vi "fgv_txtfile.vi"(7 "cmd":enum16{"write", "create"}(ring), 8 "err in":errorcluster) -> (0 "error out":errorcluster caption="err out")   [LabVIEW 2016]
uses:
  <vilib>/Utility/file.llb/Write To Spreadsheet File (string).vi
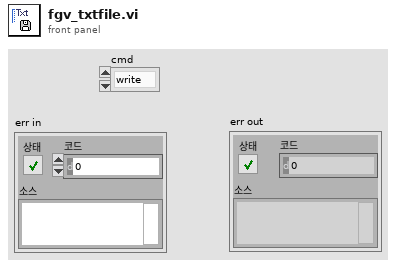
[diagram p1: front panel]
types:
  T1 = enum16{"open", "replace", "create", "open or create", "replace or create", "replace or create with confirmation"}
  T2 = typedef "Total data.ctl" = cluster{"Raw Data":T3, "Resister result data":T4, "Result Table update":cluster{"Num":u32[], "Resister 1~5":u8[][], "Resister 6~10":u8[][], "Resister 11~15":u8[][]}, "Strain Data":cluster{"Strain 1":dbl, "Strain 2":dbl, "Strain 3":dbl, "Strain 4":dbl}, "Acc Result":cluster{"Acc Peak":dbl, "Acc time":dbl, "Acc area":dbl}, "STATUS":cluster{"status":string, "all_fail":bool, "emg":bool, "cycle":u16, "file name":string}, "Speed":dbl, "Acc peak time":dbl, "Max Strain":dbl, "Resistor at peak":cluster{"[0]":dbl, "[1]":dbl, "[2]":dbl, "[3]":dbl, "[4]":dbl, "[5]":dbl, "[6]":dbl, "[7]":dbl, "[8]":dbl, "[9]":dbl, "[10]":dbl, "[11]":dbl, "[12]":dbl, "[13]":dbl, "[14]":dbl}, "Acc peak index":u32, "time":string, "Cycle finish":bool, "Resistor at ini":cluster{"[0]":dbl, "[1]":dbl, "[2]":dbl, "[3]":dbl, "[4]":dbl, "[5]":dbl, "[6]":dbl, "[7]":dbl, "[8]":dbl, "[9]":dbl, "[10]":dbl, "[11]":dbl, "[12]":dbl, "[13]":dbl, "[14]":dbl}}
  T3 = typedef "raw Q data.ctl" = cluster{"Res_data":waveform(dbl)[], "Acc_data":waveform(dbl), "Strain_data":waveform(dbl)[]}
  T4 = typedef "raw data type.ctl" = cluster{"Resistor values":cluster{"[0]":dbl, "[1]":dbl, "[2]":dbl, "[3]":dbl, "[4]":dbl, "[5]":dbl, "[6]":dbl, "[7]":dbl, "[8]":dbl, "[9]":dbl, "[10]":dbl, "[11]":dbl, "[12]":dbl, "[13]":dbl, "[14]":dbl}, "Resistor tables":u8[], "Pass Fails":bool[]}
  T5 = cluster{"Strain 1":dbl, "Strain 2":dbl, "Strain 3":dbl, "Strain 4":dbl}
  T6 = cluster{"[0]":dbl, "[1]":dbl, "[2]":dbl, "[3]":dbl, "[4]":dbl, "[5]":dbl, "[6]":dbl, "[7]":dbl, "[8]":dbl, "[9]":dbl, "[10]":dbl, "[11]":dbl, "[12]":dbl, "[13]":dbl, "[14]":dbl}
  T7 = cluster{"Test Information":cluster{"date":string, "custom":string, "oper":string, "package":string, "pkg side":string, "solder":string, "brd side":string, "paste":string, "reflow":string}, "Sensor Set":cluster{"Accelerometer":cluster{"Sensitivity(mV/g)":dbl}, "Strain Guage":cluster{"Ch.":dbl[], "Gage factor":dbl[], "Resistance":dbl[], "Poisson ratio":dbl[]}}, "Resistor Set":cluster{"Criterion Level":dbl, "Res. Set":cluster{"Res. Ch":dbl, "Res. Active":bool, "Res Initial":dbl}[]}, "Test Stop Condition":cluster{"Test cycle":u16, "Fail number in a cycle":u16, "Fail factor":cluster{"Duration":u16, "Fail No.":u16}}, "Acceleration Condition ":cluster{"Shock duration pecent [%]":u16, "Filter cutoff freq":u32}, "Save":cluster{"Save Path":path, "File Name":string}}
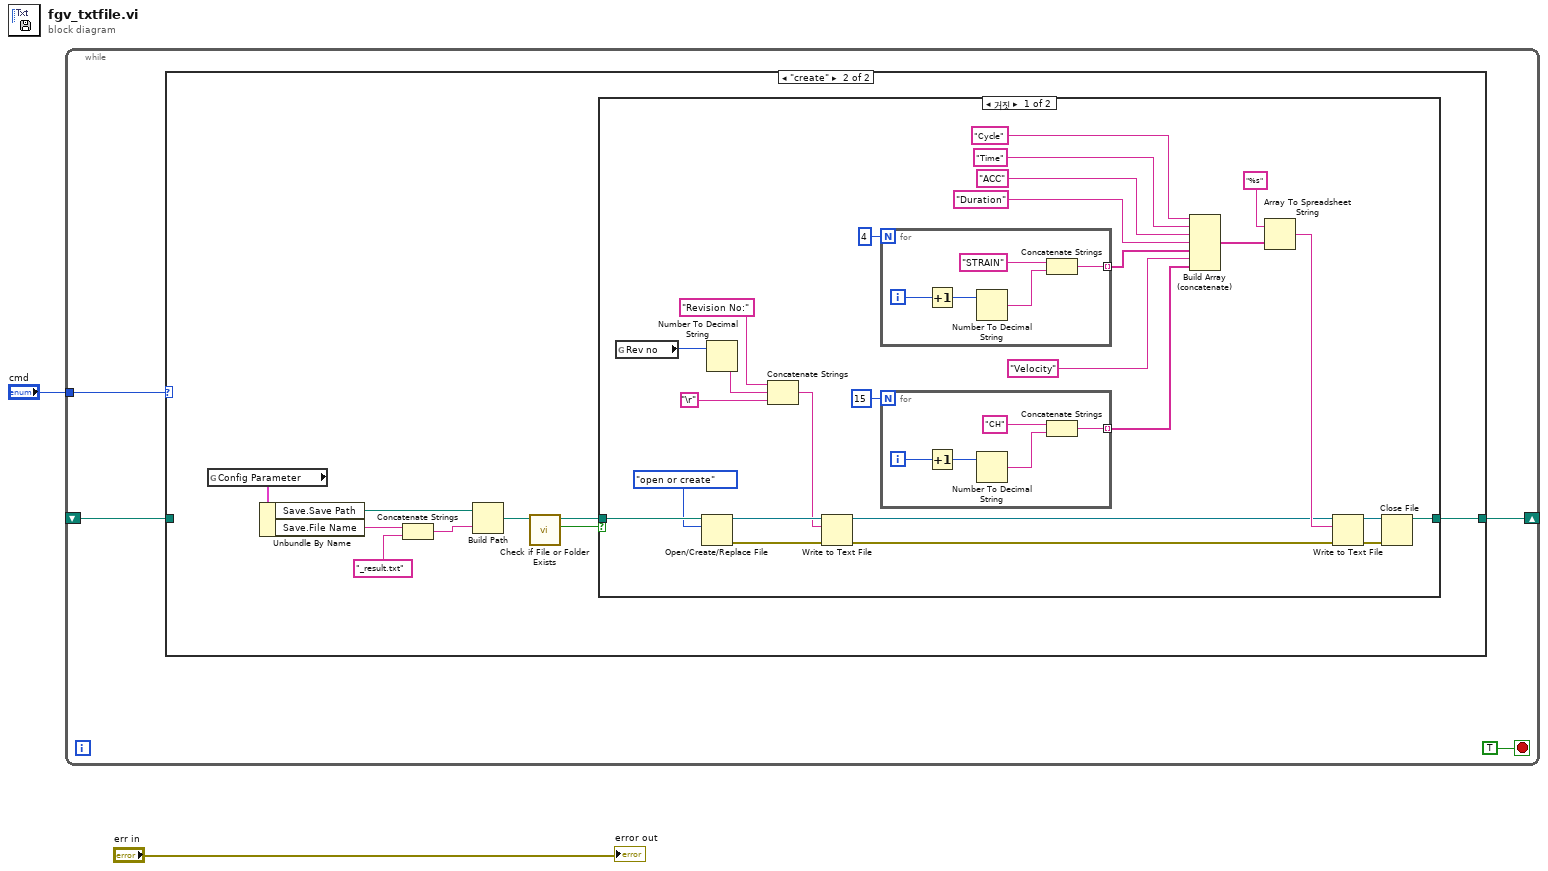
[diagram p0: block diagram]
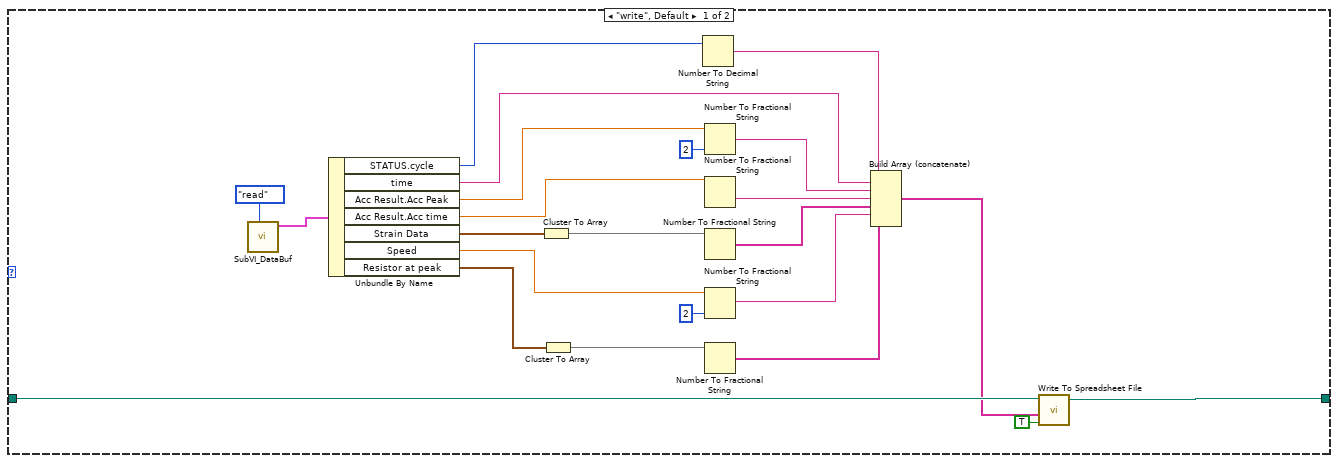
[diagram p2: hidden frame]
diagram:
  n1 = while {
    tunnel: "cmd" -> [w5]
    shift-right: [w4] -> _
    shift-left: _ -> [w3]
    stop <- TRUE stop-if-true
    n2 = case shown="\"create\"" w5 {
      tunnel: [w28 w30] -> w4
      tunnel: w3 -> [w25 _]
      frame "write", Default {
        n3 = call "SubVI_DataBuf.vi"("cmd"=enum16{"ini", "write", "read"}."read") -> ("Total data 2"=w27:T2)  [unwired: 9 in, 1 out]
        n4 = Unbundle By Name(w27) -> ("STATUS.cycle"=w24:u16, "time"=w7:string, "Acc Result.Acc Peak"=w23:dbl, "Acc Result.Acc time"=w9:dbl, "Strain Data"=w21:T5, "Speed"=w11:dbl, "Resistor at peak"=w13:T6)
        n5 = Cluster To Array(cluster=w21) -> (array=w20:dbl[])
        n6 = Cluster To Array(cluster=w13) -> (array=w19:dbl[])
        n7 = Number To Decimal String(number=w24) -> (decimal integer string=w18:string)  [unwired: 1 in]
        n8 = Number To Fractional String(number=w23, precision (6)=i16 2 ("정밀도(6)")) -> (F-format string=w17:string)  [unwired: 2 in]
        n9 = Number To Fractional String(number=w9) -> (F-format string=w8:string)  [unwired: 3 in]
        n10 = Number To Fractional String(number=w20) -> (F-format string=w16:string[])  [unwired: 3 in]
        n11 = Number To Fractional String(number=w11, precision (6)=i16 2 ("정밀도(6)")) -> (F-format string=w10:string)  [unwired: 2 in]
        n12 = Number To Fractional String(number=w19) -> (F-format string=w15:string[])  [unwired: 3 in]
        n13 = Build Array (concatenate)(w18, w7, w17, w8, w16, w10, w15) -> (w14:string[])
        n14 = call-poly <vilib>:"Write To Spreadsheet File.vi"("append to file? (new file:F)"=TRUE, "1D data"=w14, "file path (dialog if empty)"=w25) -> ("new file path (Not A Path if cancelled)"=w28:path)  [unwired: 5 in]
      }
      frame "create" {
        n15 = global read "글로벌_Config Parameter.vi" "Config Parameter"() -> (w34:T7)
        n16 = Unbundle By Name(w34) -> ("Save.Save Path"=w35:path, "Save.File Name"=w37:string)
        n17 = Concatenate Strings(w37, "_result.txt" ("문자열")) -> (w38:string)
        n18 = Build Path(base path=w35, name or relative path=w38) -> (appended path=w33:path)
        n19 = call <vilib>:"Check if File or Folder Exists.vi"("path"=w33) -> ("file or folder exists?"=w32:bool, "dup path"=w31:path)  [unwired: 8 in, 1 out]
        n20 = case shown="거짓" w32 {
          tunnel: w31 -> [w64 w75]
          tunnel: [w62 w75] -> w30
          frame False {
            n21 = global read "글로벌_Config Parameter.vi" "Rev no"() -> (w43:u32)
            n22 = Open/Create/Replace File(file path (use dialog)=w64, operation (0:open)=T1."open or create" ("동작(0:open)")) -> (refnum out=w47:refnum<file>, error out=w46:errorcluster)  [unwired: 4 in, 1 out]
            n23 = Number To Decimal String(number=w43) -> (decimal integer string=w42:string)  [unwired: 1 in]
            n24 = Concatenate Strings("Revision No:" ("문자열"), w42, "\r") -> (w39:string)
            n25 = Write to Text File(file (use dialog)=w47, text=w39, error in=w46) -> (refnum out=w44:refnum<file>, error out=w45:errorcluster)  [unwired: 1 in, 1 out]
            n26 = for {
              N: 4 -> [_]
              tunnel: [w65] -> w56 mode=indexing
              i -> [w68]
              n27 = Increment(x=w68) -> (x+1=w69:i32)
              n28 = Number To Decimal String(number=w69) -> (decimal integer string=w67:string)  [unwired: 1 in]
              n29 = Concatenate Strings("STRAIN" ("문자열"), w67) -> (w65:string)
            }
            n30 = for {
              N: 15 -> [_]
              tunnel: [w70] -> w55 mode=indexing
              i -> [w73]
              n31 = Increment(x=w73) -> (x+1=w74:i32)
              n32 = Number To Decimal String(number=w74) -> (decimal integer string=w72:string)  [unwired: 1 in]
              n33 = Concatenate Strings("CH" ("문자열"), w72) -> (w70:string)
            }
            n34 = Build Array (concatenate)("Cycle" ("문자열"), "Time" ("문자열"), "ACC" ("문자열"), "Duration" ("문자열"), w56, "Velocity" ("문자열"), w55) -> (w58:string[])
            n35 = Array To Spreadsheet String(array=w58, 3:"%s" ("포맷 문자열")) -> (spreadsheet string=w52:string)  [unwired: 1 in]
            n36 = Write to Text File(file (use dialog)=w44, text=w52, error in=w45) -> (refnum out=w61:refnum<file>, error out=w60:errorcluster)  [unwired: 1 in, 1 out]
            n37 = Close File(refnum=w61, error in=w60) -> (path=w62:path)  [unwired: 1 out]
          }
          frame True {
          }
        }
      }
    }
  }
  "error out" <- "err in"
